vi "Drive_Utils_UpdatePosition.vi"(0 "delta right":dbl, 1 "delta left":dbl, 2 "speed left":dbl, 3 "speed right":dbl, 4 "error in (no error)":errorcluster) -> (5 "state out":T1, 6 "error out":errorcluster)   [LabVIEW 2009, in "Drive.lvlib" / "Drive_Utils.lvlib"]
uses:
  Drive_Utils.lvlib
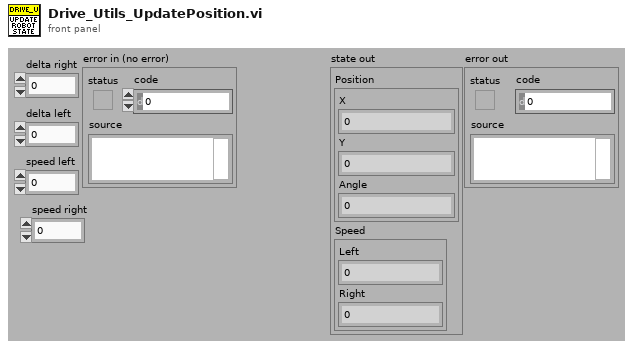
[diagram p1: front panel]
types:
  T1 = cluster{"Position":cluster{"X":dbl, "Y":dbl, "Angle":dbl}, "Speed":cluster{"Left":dbl, "Right":dbl}}
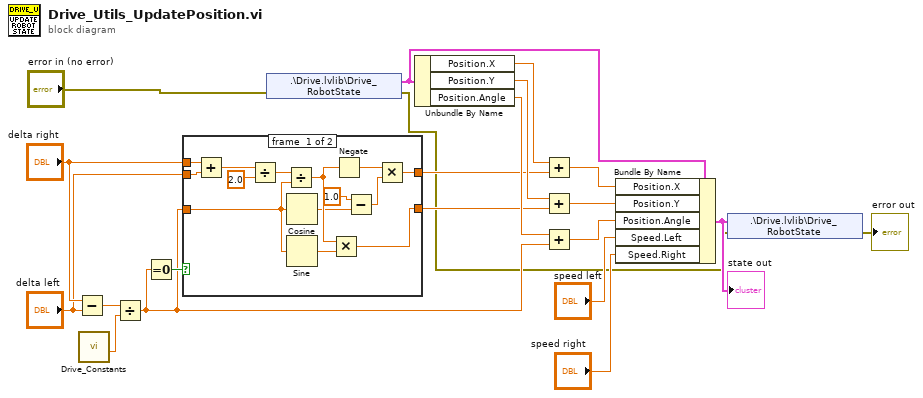
[diagram p0: block diagram]
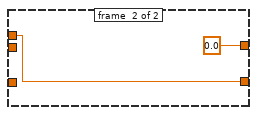
[diagram p2: hidden frame]
diagram:
  n1 = Subtract(x="delta right", y="delta left") -> (x-y=w18:dbl)
  n2 = call "Drive_Constants.vi"() -> ("Wheels interval"=w17:dbl)  [unwired: 1 in, 3 out]
  n3 = Divide(x=w18, y=w17) -> (x/y=w11:dbl)
  n4 = Equal To 0?(x=w11) -> (x = 0?=w14:bool)
  n5 = case shown="False" w14 {
    tunnel: "delta right" -> [w35 w37]
    tunnel: "delta left" -> [w34 _]
    tunnel: w11 -> [w27 _]
    tunnel: [w22 0.0 ("delta right")] -> w6
    tunnel: [w29 w37] -> w5
    frame #0 {
      n6 = Add(x=w35, y=w34) -> (x+y=w33:dbl)
      n7 = Divide(x=w33, y=2.0) -> (x/y=w31:dbl)
      n8 = Divide(x=w31, y=w27) -> (x/y=w28:dbl)
      n9 = Cosine(x=w27) -> (cos(x)=w26:dbl)
      n10 = Sine(x=w27) -> (sin(x)=w30:dbl)
      n11 = Multiply(x=w28, y=w30) -> (x*y=w29:dbl)
      n12 = Negate(x=w28) -> (-x=w24:dbl)
      n13 = Subtract(x=1.0, y=w26) -> (x-y=w23:dbl)
      n14 = Multiply(x=w24, y=w23) -> (x*y=w22:dbl)
    }
    frame #1 {
    }
  }
  n15 = shared-variable ".\\Drive.lvlib\\Drive_RobotState"(error in="error in (no error)") -> (w19:T1, error out=w2:errorcluster)
  n16 = Unbundle By Name(w19) -> ("Position.X"=w10:dbl, "Position.Y"=w8:dbl, "Position.Angle"=w16:dbl)
  n17 = Add(x=w10, y=w6) -> (x+y=w9:dbl)
  n18 = Add(x=w8, y=w5) -> (x+y=w7:dbl)
  n19 = Add(x=w16, y=w11) -> (x+y=w15:dbl)
  n20 = Bundle By Name(cluster=w19, "Position.X"=w9, "Position.Y"=w7, "Position.Angle"=w15, "Speed.Left"="speed left", "Speed.Right"="speed right") -> (w4:T1)
  "state out" <- w4
  n21 = shared-variable ".\\Drive.lvlib\\Drive_RobotState"(w4, error in=w2) -> (error out=→"error out":errorcluster)
